vi "CreateTrackingWorkingImages.vi"(8 "error in (no error)":errorcluster) -> (0 "error out":errorcluster, 3 "Tracking Images":T1)   [LabVIEW 2017, in "ImageAcquisitionLibrary.lvlib"]
uses:
  ImageAcquisitionLibrary.lvlib
  TrackingImages.ctl
  <vilib>/vision/Image Controls.llb/IMAQ Image.ctl
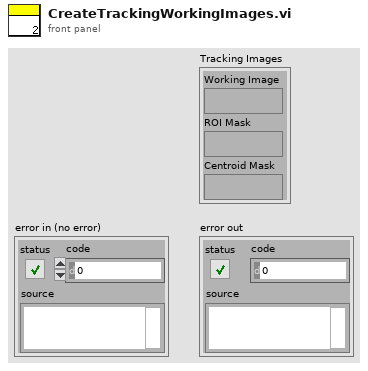
[diagram p1: front panel]
types:
  T1 = typedef "ImageAcquisitionLibrary.lvlib/TrackingImages.ctl" = cluster{"Working Image":T2, "ROI Mask":T2, "Centroid Mask":T2}
  T2 = typedef "IMAQ Image.ctl" = refnum<image>
  T3 = typedef "Image Type" = u32
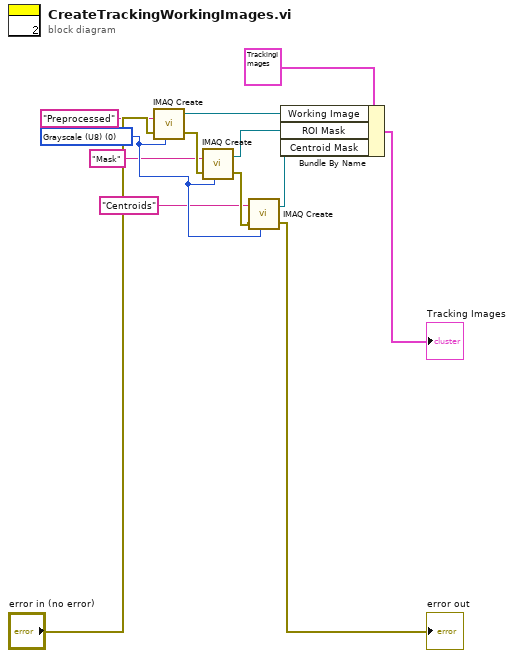
[diagram p0: block diagram]
diagram:
  w13 = T3 0 items=["Grayscale (U8)", "Grayscale (I16)", "Grayscale (SGL)", "Complex (CSG)", "RGB (U32)", "HSL (U32)", "RGB (U64)", "Grayscale (U16)"] ("Image Type")
  n1 = call "IMAQ Create"("Image Name"="Preprocessed", "Image Type"=w13, "error in (no error)"="error in (no error)") -> ("New Image"=w5:T2, "error out"=w6:errorcluster)  [unwired: 2 in]
  n2 = call "IMAQ Create"("Image Name"="Mask", "Image Type"=w13, "error in (no error)"=w6) -> ("New Image"=w4:T2, "error out"=w10:errorcluster)  [unwired: 2 in]
  n3 = call "IMAQ Create"("Image Name"="Centroids", "Image Type"=w13, "error in (no error)"=w10) -> ("New Image"=w12:T2, "error out"=→"error out":errorcluster)  [unwired: 2 in]
  n4 = Bundle By Name(cluster=T1 {"Working Image"=refnum, "ROI Mask"=refnum, "Centroid Mask"=refnum}, "Working Image"=w5, "ROI Mask"=w4, "Centroid Mask"=w12) -> (→"Tracking Images":T1)
